vi "CreatePrivateEvents.vi"(8 "error in (no error)":errorcluster, 11 "Inst.Attocube-3DR":refnum<class "Inst.Attocube-3DR.lvclass">) -> (0 "error out":errorcluster, 3 "Inst.Attocube-3DR out":refnum<class "Inst.Attocube-3DR.lvclass">)   [LabVIEW 2019, in "Inst.Attocube-3DR.lvclass"]
doc: "---------------------------------------------------------------\nJKI State Machine Objects™\nhttp://jki.net/state-machine-objects/\nCopyright (C) 2005-2015, JKI <info@jki.net>\nALL RIGHTS RESERVEDJKI State Machine Objects (SMO) 1.0.0.4\nJKI - JKI\nCopyright (c) 2015, JKI"
uses:
  Inst.Attocube-3DR.lvclass
  Typedefs/PrivateEvents--Inst.Attocube-3DR.MessageToProcess.ctl
  <userlib>/LevyLab/Instrument Framework/SMOs/RemoteControl/Typedefs/Message--Cluster.ctl
  Inst.Attocube-3DR.lvclass/Inst.Attocube-3DR.ctl
  <userlib>/LevyLab/Instrument Framework/Instrument Types/VSource/Instrument.VSource.lvclass
  <userlib>/LevyLab/Instrument Framework/SMOs/RemoteControl/RemoteControl.lvclass
panel:
  # "For instructions on how to use the JKI State Machine Objects, examples and video tutorials, visit:\nhttp://jki.net/state-machine-objects/\n\nJKI State Machine Objects™\nhttp://jki.net/state-machine-objects/\nCopyright (C) 2005-2015, JKI <info@jki.net>\nALL RIGHTS RESERVED"
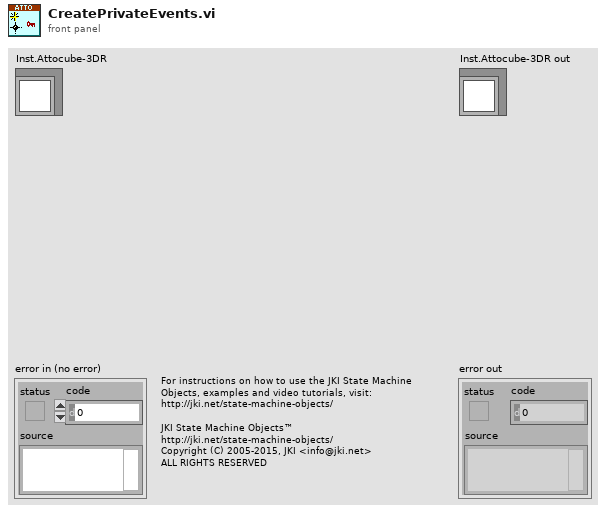
[diagram p1: front panel]
types:
  T1 = typedef "Inst.Attocube-3DR.lvclass/PrivateEvents--Inst.Attocube-3DR.MessageToProcess.ctl" = cluster{"Message":T2}
  T2 = typedef "RemoteControl.lvclass/Message--Cluster.ctl" = cluster{"Command":string, "Data":variant, "ID":string}
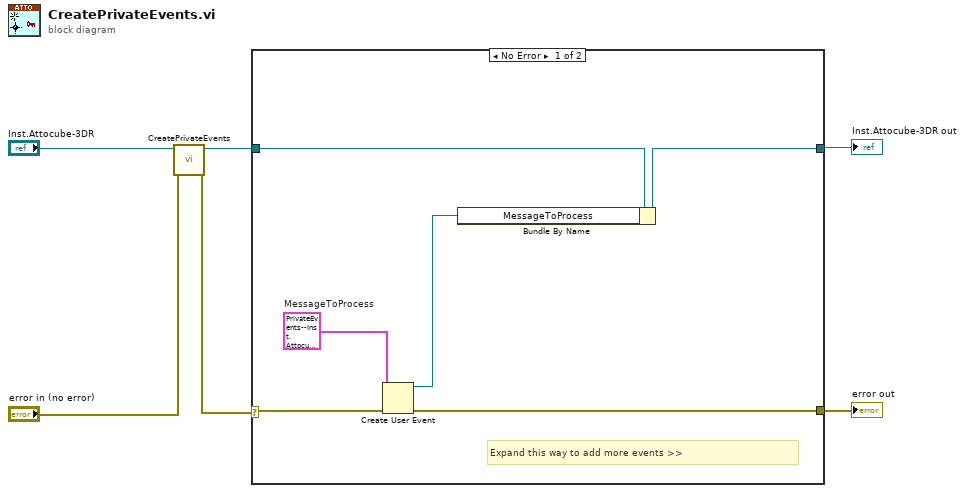
[diagram p0: block diagram]
diagram:
  n1 = call-parent "CreatePrivateEvents.vi"("error in (no error)"="error in (no error)", "Instrument"="Inst.Attocube-3DR") -> ("error out"=w1:errorcluster, "Instrument out"=w5:refnum<class "Inst.Attocube-3DR.lvclass">)  [unwired: 8 in]
  n2 = case shown="No Error" w1 {
    selector: w1 -> [w9 w14]
    tunnel: [w7 w14] -> w3
    tunnel: [w11 w13] -> w4
    tunnel: w5 -> [w12 w13]
    frame No Error {
      w10 = T1 {"Message"={"Command"="", "Data"=variant(string ""), "ID"=""}}  # MessageToProcess
      # "Expand this way to add more events >>"
      n3 = Create User Event(user event datatype=w10, error in=w9) -> (user event=w8:refnum<user-event>, error out=w7:errorcluster)
      n4 = Bundle By Name(cluster=w12, "MessageToProcess"=w8) -> (w11:refnum<class "Inst.Attocube-3DR.lvclass">)
    }
    frame Error {
    }
  }
  "error out" <- w3
  "Inst.Attocube-3DR out" <- w4
